vi "result_ready.vi"(8 "error in (no error)":errorcluster, 11 "result_from_call in":refnum<class "result_from_call.lvclass">) -> (0 "error out":errorcluster, 2 "is":bool, 3 "result_from_call out":refnum<class "result_from_call.lvclass">)   [LabVIEW 2015, in "result_from_call.lvclass"]
uses:
  result_from_call.lvclass
  result_from_call.lvclass/result_from_call.ctl
  result.lvclass
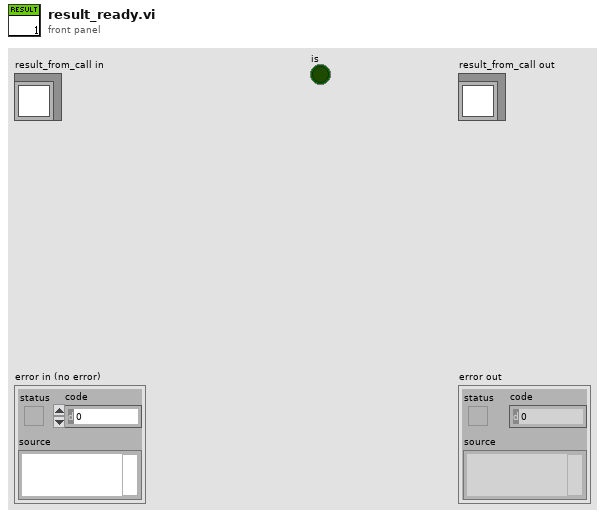
[diagram p1: front panel]
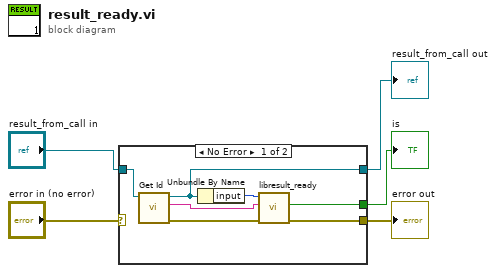
[diagram p0: block diagram]
diagram:
  n1 = case shown="No Error" "error in (no error)" {
    selector: "error in (no error)" -> [_ w14]
    tunnel: [w7 w14] -> w4
    tunnel: [w11 w13] -> w2
    tunnel: "result_from_call in" -> [w12 w13]
    tunnel: [w6 _] -> w1
    frame No Error {
      n2 = call "Get Id.vi"("result in"=w12) -> ("error out"=w10:errorcluster, "id"=w8:string, "result out"=w11:refnum<class "result_from_call.lvclass">)  [unwired: 8 in]
      n3 = Unbundle By Name(w11) -> ("input"=w9:i32)
      n4 = call "libresult_ready.vi"("error in (no error)"=w10, "id"=w8, "input"=w9) -> ("error out"=w7:errorcluster, "is"=w6:bool)  [unwired: 7 in]
    }
    frame Error {
    }
  }
  "error out" <- w4
  "result_from_call out" <- w2
  "is" <- w1
